vi "TestAdm_DateAndTimeString.vi"() -> (16 "String out":string)   [LabVIEW 2017]
doc: "Creates a time string of the format YYYY-DD-MM_HH_MM_SS\n\nThis useful in filnames etc."
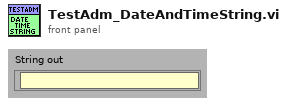
[diagram p1: front panel]
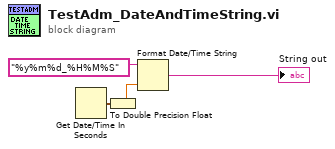
[diagram p0: block diagram]
diagram:
  n1 = Get Date/Time In Seconds() -> (seconds since 1Jan1904=w1:timestamp)
  n2 = To Double Precision Float(number=w1) -> (double precision float=w3:dbl)
  n3 = Format Date/Time String(time format string (%c)="%y%m%d_%H%M%S", seconds (now)=w3) -> (date/time string=→"String out":string)  [unwired: 1 in]
